vi "Averaging Filter.vi"(7 "Filter Size":i8, 11 "Input":dbl) -> (3 "Output":dbl)   [LabVIEW 2012]
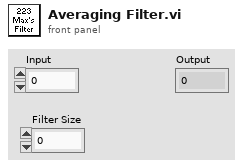
[diagram p1: front panel]
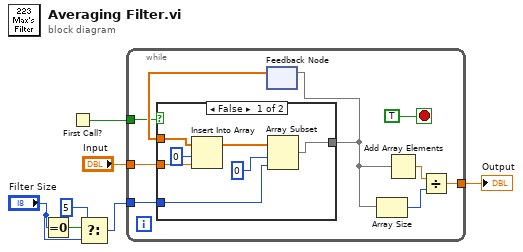
[diagram p0: block diagram]
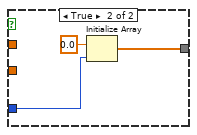
[diagram p2: hidden frame]
diagram:
  n1 = Equal To 0?(x="Filter Size") -> (x = 0?=w4:bool)
  n2 = First Call?() -> (First Call?: T/F=w5:bool)
  n3 = Select(t=i8 5, s=w4, f="Filter Size") -> (s? t:f=w2:i8)
  n4 = while {
    tunnel: w2 -> [w15]
    tunnel: "Input" -> [w14]
    tunnel: [w11] -> w6
    tunnel: w5 -> [w8]
    stop <- TRUE stop-if-true
    n5 = feedback #1() -> (w9:dbl[])  [unwired: 1 in]
    n6 = case shown="False" w8 {
      tunnel: w15 -> [w19 w25]
      tunnel: w14 -> [w23 _]
      tunnel: [w18 w24] -> w10
      tunnel: w9 -> [w17 _]
      frame False {
        n7 = Insert Into Array(array=w17, index=0, new element=w23) -> (w21:dbl[])
        n8 = Array Subset(array=w21, index=0 ("length"), length=w19) -> (w18:dbl[])
      }
      frame True {
        n9 = Initialize Array(0.0 ("element"), w25) -> (w24:dbl[])
      }
    }
    n10 = feedback-in #1(w10) -> ()
    n11 = Array Size(array=w10) -> (size(s)=w13:i32)
    n12 = Add Array Elements(numeric array=w10) -> (sum=w12:dbl)
    n13 = Divide(x=w12, y=w13) -> (x/y=w11:dbl)
  }
  "Output" <- w6
